vi "BallShear_PackageCheck.vi"(11 "Power":bool) -> (3 "Ready":bool)   [LabVIEW 2013]
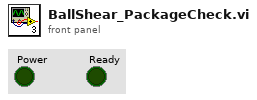
[diagram p1: front panel]
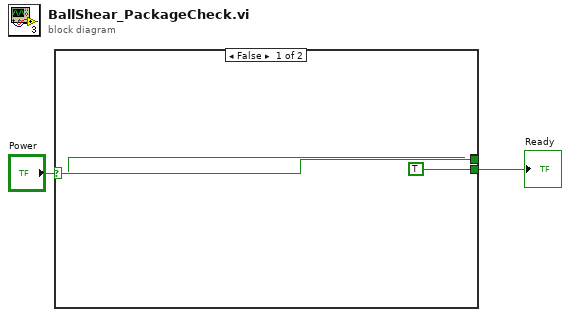
[diagram p0: block diagram]
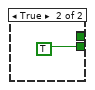
[diagram p2: hidden frame]
diagram:
  n1 = case shown="False" "Power" {
    selector: "Power" -> [w3 _]
    tunnel: [w3 w6] -> _
    tunnel: "Power" -> [_ w6]
    tunnel: [TRUE ("Power") TRUE ("Power")] -> w1
    frame False {
    }
    frame True {
    }
  }
  "Ready" <- w1
